vi "RefractiveBBO.vi"() -> ()   [LabVIEW 2019]
panel:
  out "n extraordinary":dbl
  out "n ordinary":dbl
  in  "wavelength (nm)":dbl
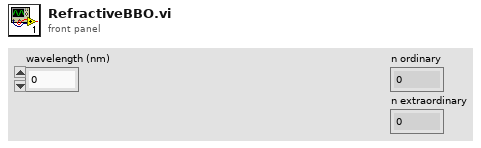
[diagram p1: front panel]
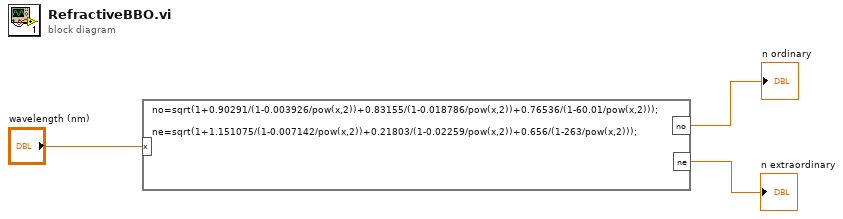
[diagram p0: block diagram]
diagram:
  n1 = formula code="no=sqrt(1+0.90291/(1-0.003926/pow(x,2))+0.83155/(1-0.018786/pow(x,2))+0.76536/(1-60.01/pow(x,2)));\n\nne=sqrt(1+1.151075/(1-0.007142/pow(x,2))+0.21803/(1-0.02259/pow(x,2))+0.656/(1-263/pow(x,2)));"("x"="wavelength (nm)") -> ("no"=→"n ordinary":dbl, "ne"=→"n extraordinary":dbl)
